vi "XY to Cluster.vi"(1 "X Data":dbl[](array[numeric]), 2 "Y Data":dbl[](array[numeric])) -> (0 "XY Cluster Array":cluster{"Numeric":dbl, "Numeric":dbl}[](array[cluster]))   [LabVIEW 2021]
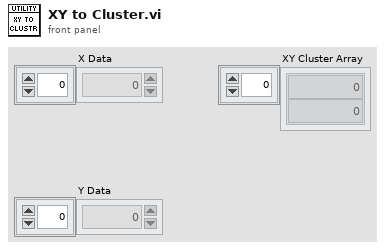
[diagram p1: front panel]
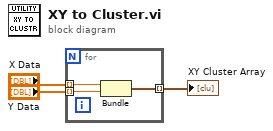
[diagram p0: block diagram]
diagram:
  n1 = for {
    tunnel: "X Data" -> [w6] mode=indexing
    tunnel: "Y Data" -> [w5] mode=indexing
    tunnel: [w4] -> w3 mode=indexing
    n2 = Bundle("Numeric"=w6, "Numeric"=w5) -> (w4:cluster{"Numeric":dbl, "Numeric":dbl})  [unwired: 1 in]
  }
  "XY Cluster Array" <- w3
